vi "Player Info.vi"(11 "third in":refnum<class "third.lvclass">) -> (0 "Defeat Speech":string, 1 "Victory Speech":string, 2 "Name":string, 3 "third out":refnum<class "third.lvclass">)   [LabVIEW 2015, in "third.lvclass"]
uses:
  third.lvclass
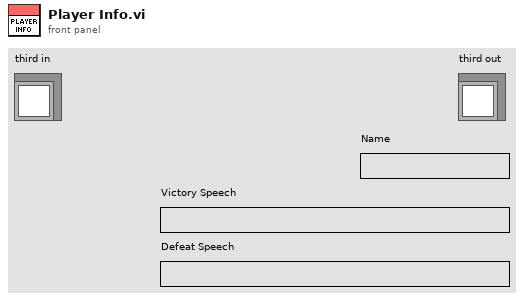
[diagram p1: front panel]
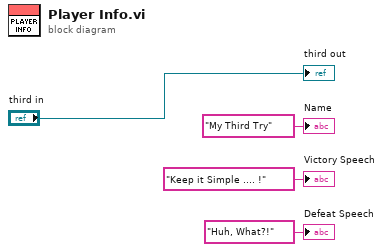
[diagram p0: block diagram]
diagram:
  "third out" <- "third in"
  "Name" <- "My Third Try" ("Name")
  "Victory Speech" <- "Keep it Simple .... !" ("Victory Speech")
  "Defeat Speech" <- "Huh, What?!" ("Defeat Speech")
